vi "AddItem__slk_tc.vi"(0 "tree control in":refnum<class "TreeControl.lvclass">, 1 "make top level? (F)":bool, 2 "child only? (F)":bool, 5 "parent tag (current tag)":string, 7 "new tag (same as text)":string, 9 "new text":string, 11 "error in (no error)":errorcluster, 12 "child position (end=-1)":i32=-1, 13 "column text {#1 and greater} (empty)":string[](array[string]), 14 "symbol (no symbol=0)":i32) -> (4 "tree control out":refnum<class "TreeControl.lvclass">, 6 "created tag":string, 15 "error out":errorcluster)   [LabVIEW 2020, in "TreeControl.lvclass"]
doc: "Adds a new item (with child only disabled) to the tree. Uses the current selection if there is no parent value input. The tag is set to the same value as the input text if it is left blank.\n<b>NOTE: TAGS MUST BE UNIQUE.</b>"
uses:
  Library/TreeControl.lvclass
  Library/TreeControl.lvclass/TreeControl.ctl
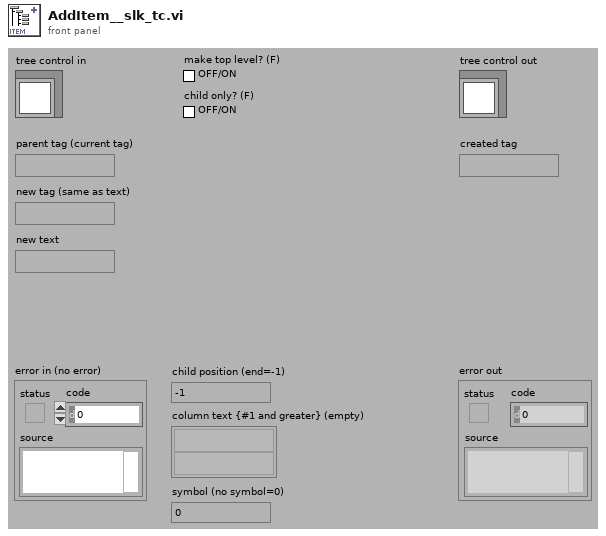
[diagram p1: front panel]
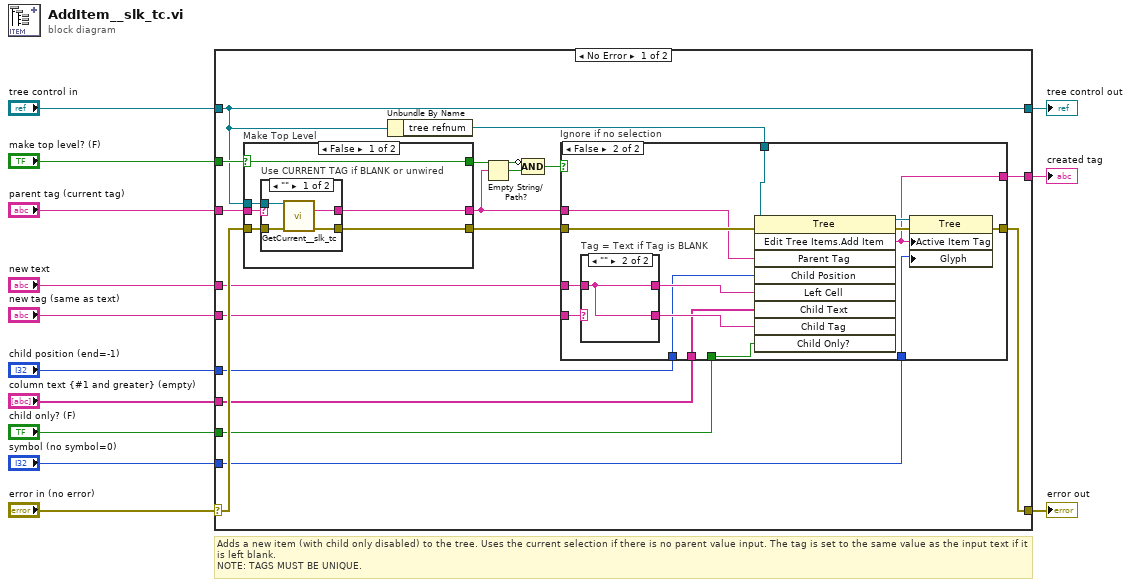
[diagram p0: block diagram]
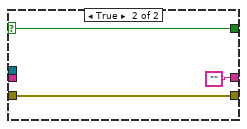
[diagram p5: hidden frame]
diagram:
  # "Adds a new item (with child only disabled) to the tree. Uses the current selection if there is no parent value input. The tag is set to the same value as the input text if it is left blank.\nNOTE: TAGS MUST BE UNIQUE."
  n1 = case shown="No Error" "error in (no error)" {
    selector: "error in (no error)" -> [w29 w67]
    tunnel: [w17 w67] -> w12
    tunnel: [w25 w66] -> w10
    tunnel: "tree control in" -> [w25 w66]
    tunnel: "make top level? (F)" -> [w31 _]
    tunnel: "parent tag (current tag)" -> [w30 _]
    tunnel: "new text" -> [w23 _]
    tunnel: "new tag (same as text)" -> [w22 _]
    tunnel: "column text {#1 and greater} (empty)" -> [w20 _]
    tunnel: "child position (end=-1)" -> [w19 _]
    tunnel: "child only? (F)" -> [w16 _]
    tunnel: [w15 _] -> w2
    tunnel: "symbol (no symbol=0)" -> [w14 _]
    frame No Error {
      n2 = case "Make Top Level" shown="False" w31 {
        selector: w31 -> [w51 w64]
        tunnel: w30 -> [w56 _]
        tunnel: w25 -> [w55 _]
        tunnel: w29 -> [w54 w65]
        tunnel: [w53 w65] -> w24
        tunnel: [w52 ""] -> w21
        tunnel: [w51 w64] -> w28
        frame False {
          n3 = case "Use CURRENT TAG if BLANK or unwired" shown="\"\"" w56 {
            selector: w56 -> [_ w62]
            tunnel: [w60 w62] -> w52
            tunnel: w55 -> [w59 _]
            tunnel: w54 -> [w58 w61]
            tunnel: [w57 w61] -> w53
            frame "" {
              n4 = call "GetCurrent__slk_tc.vi"("tree control in"=w59, "error in (no error)"=w58) -> ("current tag"=w60:string, "error out"=w57:errorcluster)  [unwired: 1 in, 11 out]
            }
            frame Default {
            }
          }
        }
        frame True {
        }
      }
      n5 = Unbundle By Name(w25) -> ("tree refnum"=w18:refnum<vi>)
      n6 = Empty String/Path?(string/path=w21) -> (empty?=w27:bool)
      n7 = Compound Arithmetic op=AND(invert w28, w27) -> (w26:bool)
      n8 = case "Ignore if no selection" shown="False" w26 {
        tunnel: w24 -> [w32 w47]
        tunnel: w23 -> [_ w45]
        tunnel: w22 -> [_ w46]
        tunnel: w21 -> [_ w44]
        tunnel: w20 -> [_ w41]
        tunnel: w19 -> [_ w38]
        tunnel: w18 -> [_ w40]
        tunnel: [w32 w36] -> w17
        tunnel: w16 -> [_ w37]
        tunnel: [_ w34] -> w15
        tunnel: w14 -> [_ w33]
        frame True {
        }
        frame False {
          n9 = case "Tag = Text if Tag is BLANK" shown="\"\"" w46 {
            selector: w46 -> [w48 _]
            tunnel: w45 -> [w49 w50]
            tunnel: [w49 w50] -> w43
            tunnel: [w48 w50] -> w42
            frame Default {
            }
            frame "" {
            }
          }
          n10 = invoke class="Tree" method="Edit Tree Items.Add Item"(reference=w40, error in=w47, "Parent Tag"=w44, "Child Position"=w38, "Left Cell"=w43, "Child Text"=w41, "Child Tag"=w42, "Child Only?"=w37) -> (reference out=w35:refnum<vi>, error out=w39:errorcluster, "Edit Tree Items:Add Item"=w34:string)  [unwired: 1 in, 6 out]
          n11 = property class="Tree"(reference=w35, error in=w39, "Active Item Tag"=w34, "Glyph"=w33) -> (error out=w36:errorcluster)  [unwired: 1 out]
        }
      }
    }
    frame Error {
    }
  }
  "error out" <- w12
  "tree control out" <- w10
  "created tag" <- w2
